vi "TimeInterpVariant_Clear.vi"(11 "in TimeInterpVariant":T1) -> (3 "out TimeInterpVariant":T1)   [LabVIEW 2019, in "Trajectory_Library.lvlib"]
doc: "Removes all samples from the history buffer.\n\nInputs:\n - In TimeInterpPose2d -- Input data cluster.\n\nOutputs:\n - Out TimeInterpPose2d -- Updated data cluster."
uses:
  Trajectory_Library.lvlib
  TypeDef/TIME_INTERPOLATABLE_VARIANT.ctl
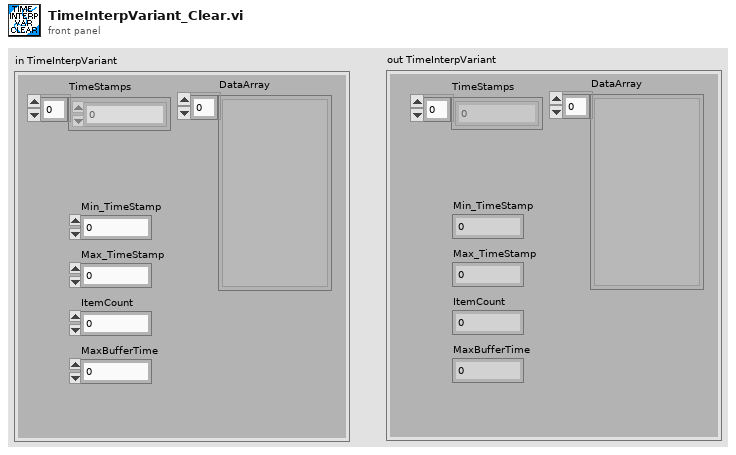
[diagram p1: front panel]
types:
  T1 = typedef "Trajectory_Library.lvlib/TIME_INTERPOLATABLE_VARIANT.ctl" = cluster{"TimeStamps":dbl[], "DataArray":variant[], "Min_TimeStamp":dbl, "Max_TimeStamp":dbl, "ItemCount":i32, "MaxBufferTime":dbl}
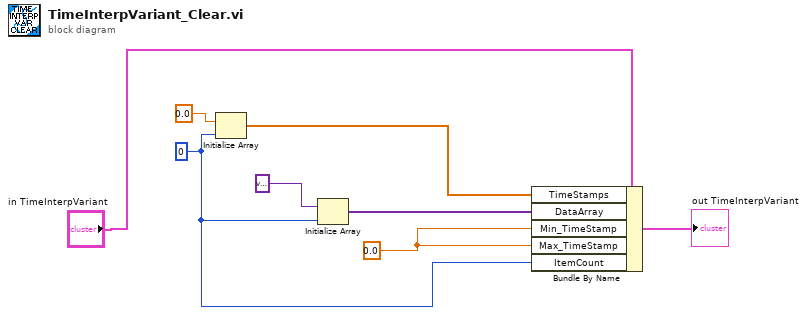
[diagram p0: block diagram]
diagram:
  w2 = 0.0 ("X")
  w1 = 0 ("dimension size")
  n1 = Initialize Array(0.0 ("element"), w1) -> (w4:dbl[])
  n2 = Initialize Array(variant ("POSE"), w1) -> (w3:variant[])
  n3 = Bundle By Name(cluster="in TimeInterpVariant", "TimeStamps"=w4, "DataArray"=w3, "Min_TimeStamp"=w2, "Max_TimeStamp"=w2, "ItemCount"=w1) -> (→"out TimeInterpVariant":T1)
